vi "run-ssh.vi"(5 "name or relative path":string="plink.exe", 6 "raw commandline":string, 7 "Remote command":string="cd /home/lvadmin/Desktop/\npwd\nmount baltic.amer.corp.natinst.com:/rnd/rnd/ /mnt/baltic\n./rtats-fix-target.sh x64 admin@10.0.86.154\n./install-greenway-io.sh /mnt/baltic/penguinExports/labviewrt/Industrial/testStack/export/3.8/3.8.0b0/ admin@10.0.86.154", 8 "error in (no error)":errorcluster, 9 "Host":string="10.0.86.122", 10 "Password":string="labview===", 11 "Username":string="root") -> (0 "error out":errorcluster, 1 "return code":i32, 2 "standard error":string, 3 "standard output":string)   [LabVIEW 2018]
uses:
  <vilib>/ErrorRing/Error Ring.xnode
  <vilib>/Utility/error.llb/Error Cluster From Error Code.vi
panel:
  out "concatenated string":string
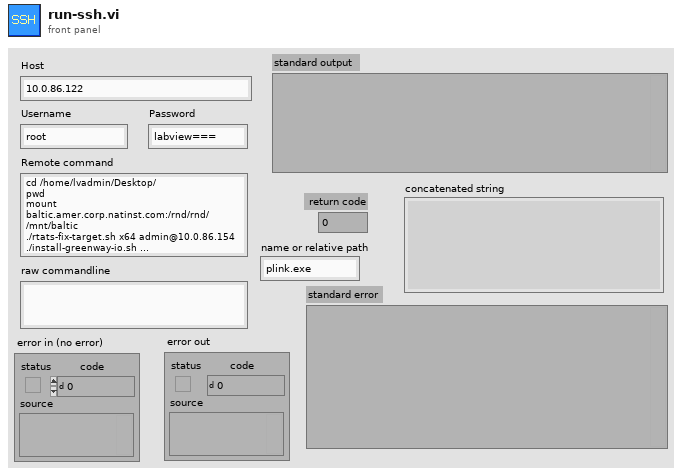
[diagram p1: front panel]
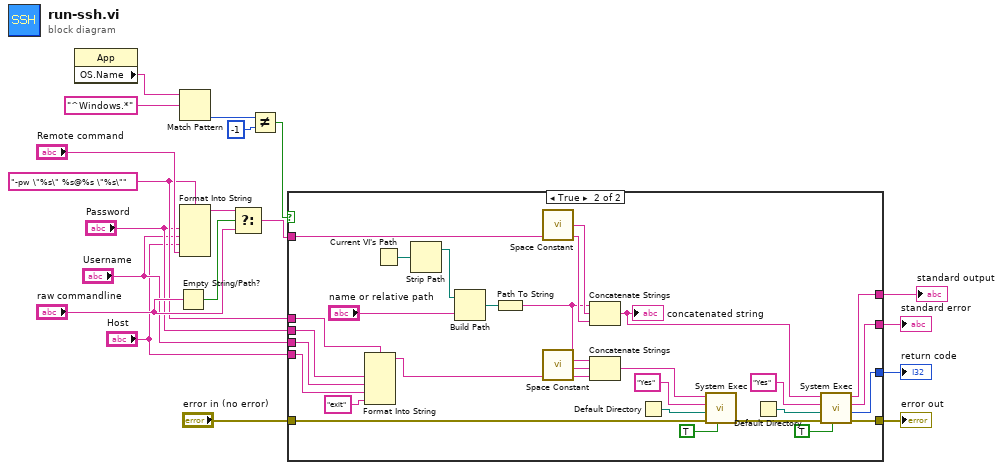
[diagram p0: block diagram]
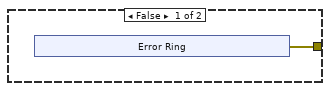
[diagram p2: hidden frame]
diagram:
  w4 = "-pw \"%s\" %s@%s \"%s\"" ("format string")
  n1 = property class="App"() -> ("OS.Name"=w11:string)  [unwired: 2 in, 2 out]
  n2 = Empty String/Path?(string/path="raw commandline") -> (empty?=w13:bool)
  n3 = Match Pattern(string=w11, regular expression="^Windows.*") -> (offset past match=w9:i32)  [unwired: 1 in, 3 out]
  n4 = Format Into String(format string=w4, "Password", "Username", "Host", "Remote command") -> (resulting string=w6:string)  [unwired: 2 in, 1 out]
  n5 = Select(t=w6, s=w13, f="raw commandline") -> (s? t:f=w12:string)
  n6 = Not Equal?(x=w9, y=-1) -> (x != y?=w7:bool)
  n7 = case shown="True" w7 {
    tunnel: "error in (no error)" -> [_ w28]
    tunnel: [_ w53] -> w18
    tunnel: [_ w52] -> w17
    tunnel: [_ w51] -> w16
    tunnel: [w20 w50] -> w15
    tunnel: w12 -> [_ w49]
    tunnel: w4 -> [_ w40]
    tunnel: "Password" -> [_ w39]
    tunnel: "Username" -> [_ w38]
    tunnel: "Host" -> [_ w37]
    frame False {
      n8 = xnode "Error Ring"() -> ("error out"=w20:errorcluster)
    }
    frame True {
      n9 = Format Into String(format string=w40, w39, w38, w37, "exit" ("input 4")) -> (resulting string=w33:string)  [unwired: 2 in, 1 out]
      n10 = Current VI's Path() -> (path=w48:path)
      n11 = Strip Path(path=w48) -> (stripped path=w47:path)  [unwired: 1 out]
      n12 = Build Path(base path=w47, name or relative path="name or relative path") -> (appended path=w43:path)
      n13 = Path To String(path=w43) -> (string=w35:string)
      n14 = call <vilib>:"Space Constant.vi"() -> ("String"=w42:string)
      n15 = call <vilib>:"Space Constant.vi"() -> ("String"=w34:string)
      n16 = Concatenate Strings(w35, w42, w49) -> (w45:string)
      "concatenated string" <- w45
      n17 = Concatenate Strings(w35, w34, w33) -> (w32:string)
      n18 = Default Directory() -> (w30:path)
      n19 = call <vilib>:"System Exec.vi"("run minimized? (F)"=TRUE, "error in (no error)"=w28, "working directory"=w30, "standard input"="Yes", "command line"=w32) -> ("error out"=w27:errorcluster)  [unwired: 3 in, 3 out]
      n20 = Default Directory() -> (w44:path)
      n21 = call <vilib>:"System Exec.vi"("run minimized? (F)"=TRUE, "error in (no error)"=w27, "working directory"=w44, "standard input"="Yes", "command line"=w45) -> ("error out"=w50:errorcluster, "return code"=w51:i32, "standard error"=w52:string, "standard output"=w53:string)  [unwired: 3 in]
    }
  }
  "standard output" <- w18
  "standard error" <- w17
  "return code" <- w16
  "error out" <- w15
